vi "SRSQCM200_subVI_V2.vi"(0 "SRS QCM init":T1, 1 "Frequency in":dbl, 2 "Gate time":u16, 3 "iteration number":i32) -> (6 "Numeric Control out":dbl, 7 "info out":T1, 8 "Frequency out 3":dbl, 9 "plot freq":T3, 10 "M,F,MR output cluster":T2)   [LabVIEW 2014]
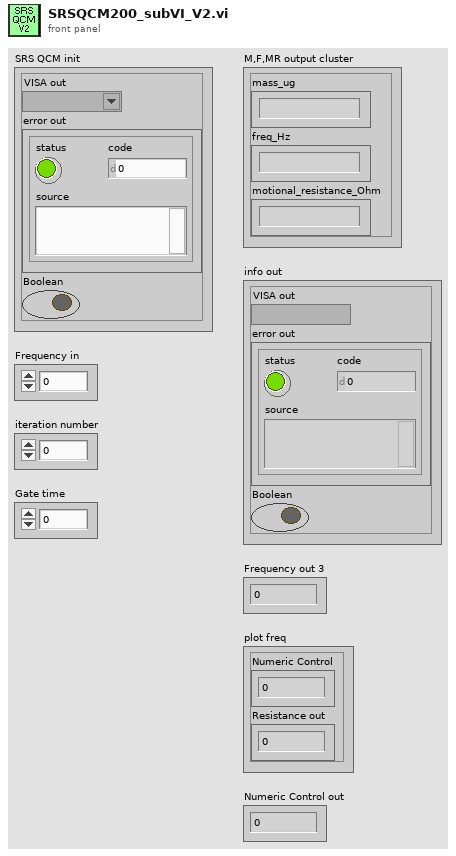
[diagram p1: front panel]
types:
  T1 = cluster{"VISA out":refnum<visa-resource-name>, "error out":errorcluster, "Boolean":bool}
  T2 = cluster{"mass_ug":string, "freq_Hz":string, "motional_resistance_Ohm":string}
  T3 = cluster{"Numeric Control":dbl, "Resistance out":dbl}
  T4 = cluster{"String":string, "String":string, "String":string}
  T5 = cluster{"VISA out":refnum<visa-resource-name>, "error out":errorcluster, bool}
  T6 = cluster{"Boolean":bool, "VISA out":refnum<visa-resource-name>, "error out":errorcluster}
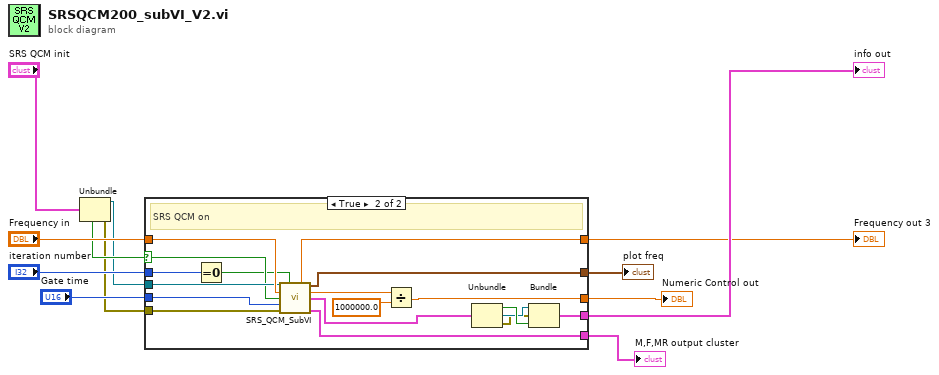
[diagram p0: block diagram]
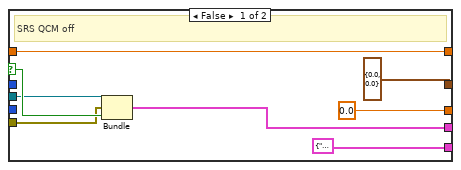
[diagram p2: hidden frame]
diagram:
  n1 = Unbundle("SRS QCM init") -> ("VISA out"=w2:refnum<visa-resource-name>, "error out"=w3:errorcluster, "Boolean"=w4:bool)
  n2 = case "SRS QCM" shown="True" w4 {
    selector: w4 -> [w20 w34]
    tunnel: w2 -> [w17 w35]
    tunnel: w3 -> [w16 w36]
    tunnel: "Frequency in" -> [w18 w38]
    tunnel: [w18 w37] -> w5
    tunnel: [T4 {"String"="", "String"="", "String"=""} ("M,F,MR output cluster") w33] -> w8
    tunnel: "iteration number" -> [_ w29]
    tunnel: [w13 w24] -> w9
    tunnel: [T3 {"Numeric Control"=0.0, "Resistance out"=0.0} ("Cluster") w23] -> w10
    tunnel: [0.0 w22] -> w11
    tunnel: "Gate time" -> [_ w21]
    frame False {
      # "SRS QCM off"
      n3 = Bundle("VISA out"=w17, "error out"=w16, w20) -> (w13:T5)  [unwired: 1 in]
    }
    frame True {
      # "SRS QCM on"
      n4 = Equal To 0?(x=w29) -> (x = 0?=w30:bool)
      n5 = call "SRS_QCM_SubVI.vi"("VISA Refnum in"=w35, "first iteration?"=w30, "Frequency out 3"=w38, "Boolean 2"=w34, "Gate time"=w21, "error in (no error)"=w36) -> ("Frequency out 2"=w37:dbl, "Cluster"=w23:T3, "Frequency out"=w31:dbl, "Cluster 2"=w28:T6, "M,F,MR output cluster"=w33:T4)  [unwired: 2 in, 3 out]
      n6 = Divide(x=w31, y=1000000.0) -> (x/y=w22:dbl)
      n7 = Unbundle(w28) -> ("Boolean"=w27:bool, "VISA out"=w26:refnum<visa-resource-name>, "error out"=w25:errorcluster)
      n8 = Bundle("VISA out"=w26, "error out"=w25, "Boolean"=w27) -> (w24:T1)  [unwired: 1 in]
    }
  }
  "Numeric Control out" <- w11
  "plot freq" <- w10
  "info out" <- w9
  "M,F,MR output cluster" <- w8
  "Frequency out 3" <- w5
